vi "Untitled 4.vi"() -> ()   [LabVIEW 2019]
panel:
  in  "b 4":bool
  out "LED 3":bool
  out "LED 2":bool
  out "LED1":bool
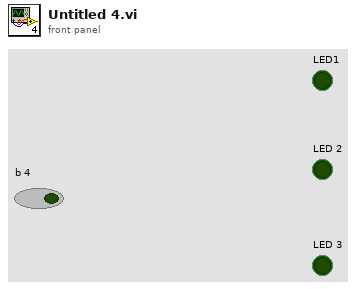
[diagram p1: front panel]
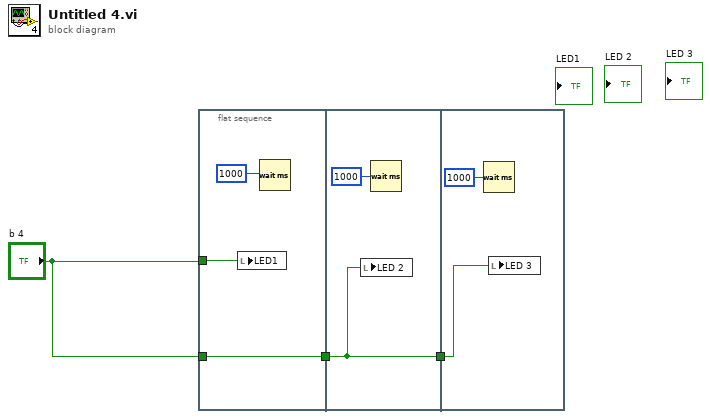
[diagram p0: block diagram]
diagram:
  n1 = flat-sequence {
    tunnel: "b 4" -> [w5]
    tunnel: [w6] -> w3
    tunnel: "b 4" -> [w6]
    tunnel: w3 -> [w8]
    tunnel: [w8] -> w2
    tunnel: w2 -> [w10]
    frame #0 {
      n2 = local write "LED1"(w5) -> ()
      n3 = Wait (ms)(milliseconds to wait=u32 1000 ("millisecond timer value")) -> ()  [unwired: 1 out]
    }
    frame #1 {
      n4 = local write "LED 2"(w8) -> ()
      n5 = Wait (ms)(milliseconds to wait=u32 1000) -> ()  [unwired: 1 out]
    }
    frame #2 {
      n6 = Wait (ms)(milliseconds to wait=u32 1000) -> ()  [unwired: 1 out]
      n7 = local write "LED 3"(w10) -> ()
    }
  }
